vi "sub_plot_single_channel.vi"(4 "Data column":dbl[](array[numeric]), 6 "Set voltage column":dbl[](array[numeric]), 8 "Cluster":cluster{dbl[], dbl[]}, 9 "Channel":i32, 10 "Front_panel_refs":T1) -> (0 "Cluster out":cluster{dbl[], dbl[]})   [LabVIEW 2016]
doc: "Creates IV/CV curve for a single channel."
uses:
  refs_front_panel.ctl
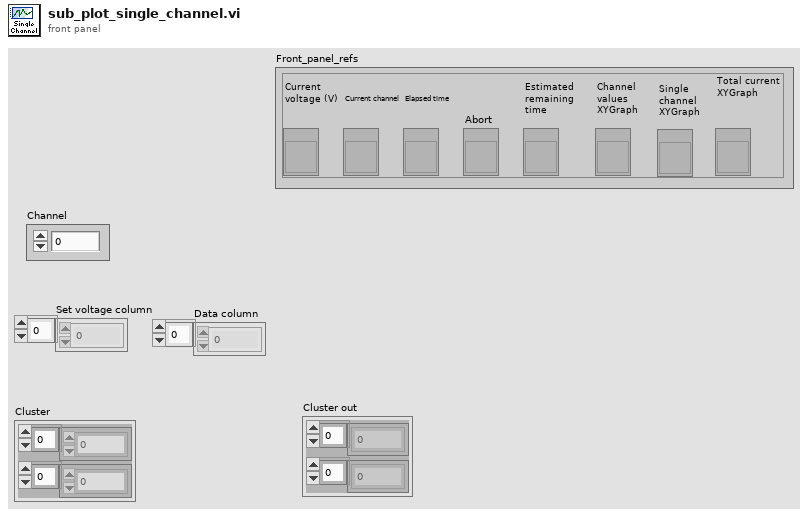
[diagram p1: front panel]
types:
  T1 = typedef "refs_front_panel.ctl" = cluster{"Current voltage (V)":refnum<vi>, "Elapsed time":refnum<vi>, "Current channel":refnum<vi>, "Abort":refnum<vi>, "Estimated remaining time":refnum<vi>, "Channel values XYGraph":refnum<vi>, "Single channel XYGraph":refnum<vi>, "Total current XYGraph":refnum<vi>}
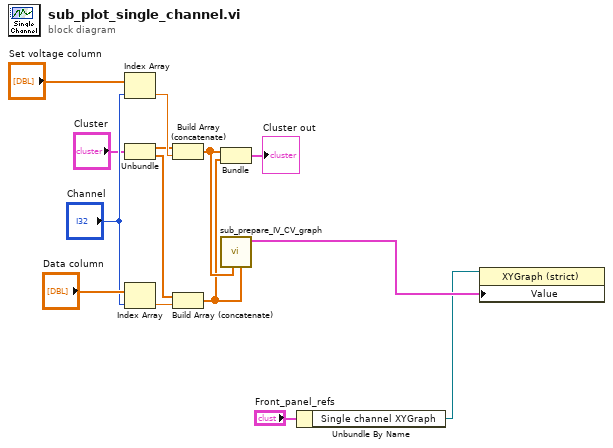
[diagram p0: block diagram]
diagram:
  n1 = Index Array(array="Set voltage column", index="Channel") -> (element=w14:dbl)
  n2 = Unbundle("Cluster") -> (w7:dbl[], w6:dbl[])
  n3 = Index Array(array="Data column", index="Channel") -> (element=w13:dbl)
  n4 = Build Array (concatenate)(w7, w14) -> (w5:dbl[])
  n5 = Build Array (concatenate)(w6, w13) -> (w4:dbl[])
  n6 = Bundle(w5, w4) -> (→"Cluster out":cluster{dbl[], dbl[]})  [unwired: 1 in]
  n7 = call "sub_prepare_IV_CV_graph.vi"("Y array"=w4, "X array"=w5) -> ("XY Graph"=w12:cluster{"X array":dbl[], "Y array":dbl[]}[])  [unwired: 9 in]
  n8 = Unbundle By Name("Front_panel_refs") -> ("Single channel XYGraph"=w1:refnum<vi>)
  n9 = property class="XYGraph (strict)"(reference=w1, "Value"=w12) -> ()  [unwired: 1 in, 2 out]
